vi "Read Sensor Scaling.vi"(0 "Cal Base Path":path) -> (4 "Sensors scaling":T1(array[cluster]))   [LabVIEW 2023]
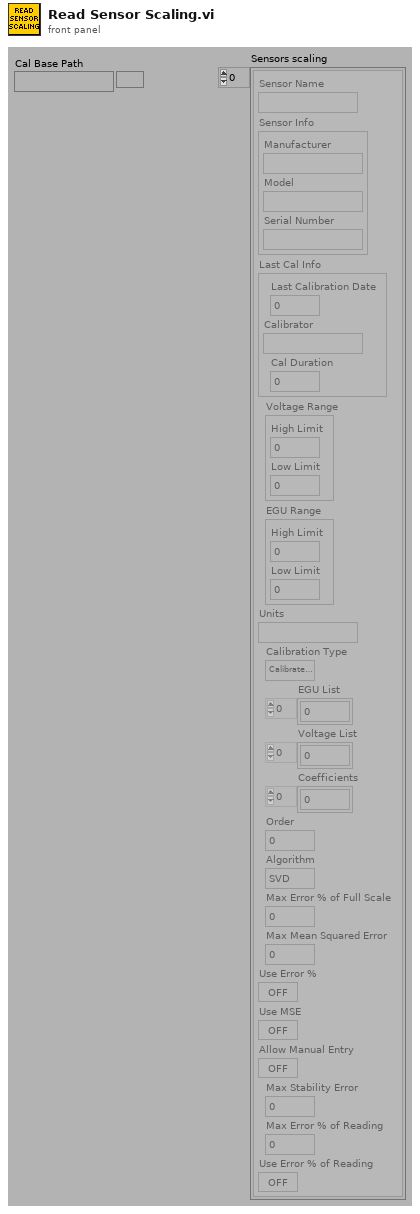
[diagram p1: front panel]
types:
  T1 = cluster{"Sensor Name":string, "Sensor Info":cluster{"Manufacturer":string, "Model":string, "Serial Number":string}, "Last Cal Info":cluster{"Last Calibration Date":dbl, "Calibrator":string, "Cal Duration":i32}, "Voltage Range":cluster{"High Limit":dbl, "Low Limit":dbl}, "EGU Range":cluster{"High Limit":dbl, "Low Limit":dbl}, "Units":string, "Calibration Type":enum16{"Calibrate Analog", "Compare Analog Calibration"}, "EGU List":dbl[], "Voltage List":dbl[], "Coefficients":dbl[], "Order":i32, "Algorithm":enum32{"SVD", "Givens", "Givens2", "Householder", "LU Decomposition", "Cholesky"}, "Max Error % of Full Scale":dbl, "Max Mean Squared Error":dbl, "Use Error %":bool, "Use MSE":bool, "Allow Manual Entry":bool, "Max Stability Error":dbl, "Max Error % of Reading":dbl, "Use Error % of Reading":bool}[]
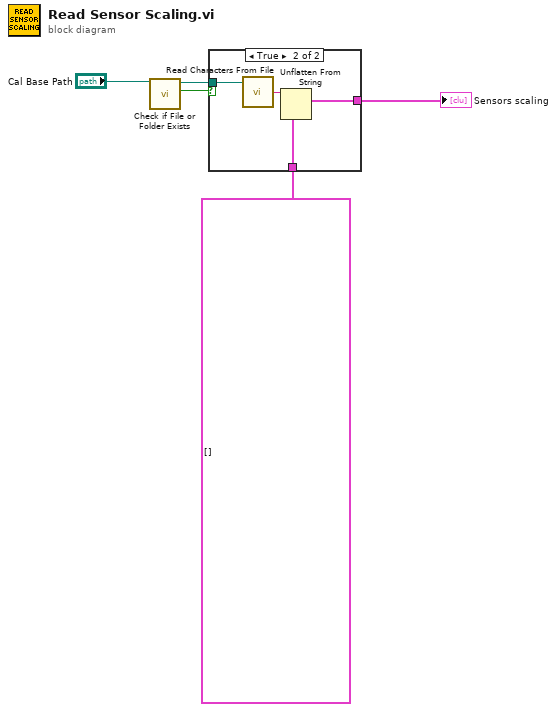
[diagram p0: block diagram]
diagram:
  n1 = call <vilib>:"Check if File or Folder Exists.vi"("path"="Cal Base Path") -> ("file or folder exists?"=w3:bool, "dup path"=w2:path)  [unwired: 8 in, 1 out]
  n2 = case shown="True" w3 {
    tunnel: T1 [] ("Sensors Info") -> [w6 w10]
    tunnel: [w6 w9] -> w4
    tunnel: w2 -> [_ w7]
    frame False {
    }
    frame True {
      n3 = call <vilib>:"Read Characters From File.vi"("file path (dialog if empty)"=w7) -> ("character string"=w8:string)  [unwired: 5 in, 3 out]
      n4 = Unflatten From String(type=w10, binary string=w8) -> (value=w9:T1)  [unwired: 3 in, 2 out]
    }
  }
  "Sensors scaling" <- w4
